vi "xiC - IMAQ - ErrorDialog.vi"(8 "error in (no error)":errorcluster, 11 "Attributes In":T1) -> (0 "error out":errorcluster, 3 "Attributes Out":T1)   [LabVIEW 2013]
uses:
  xiC - IMAQ - Attributes.ctl
  C:/Projects/Cameras3.x/xiLib/xiLIB_64bit/xiLIB/xiCamLib/API/x64/xiApi.NETX64.dll
  xiLIB_64bit/xiLIB/xiCamLib/API/x64/xiApi.NETX64.dll
  xiC - IMAQ - TreeDisplayType.ctl
  xiC - IMAQ - Globals.vi
panel:
  in  "CopyToClipboard":bool
  in  "EXIT":bool
  out "INFO":string
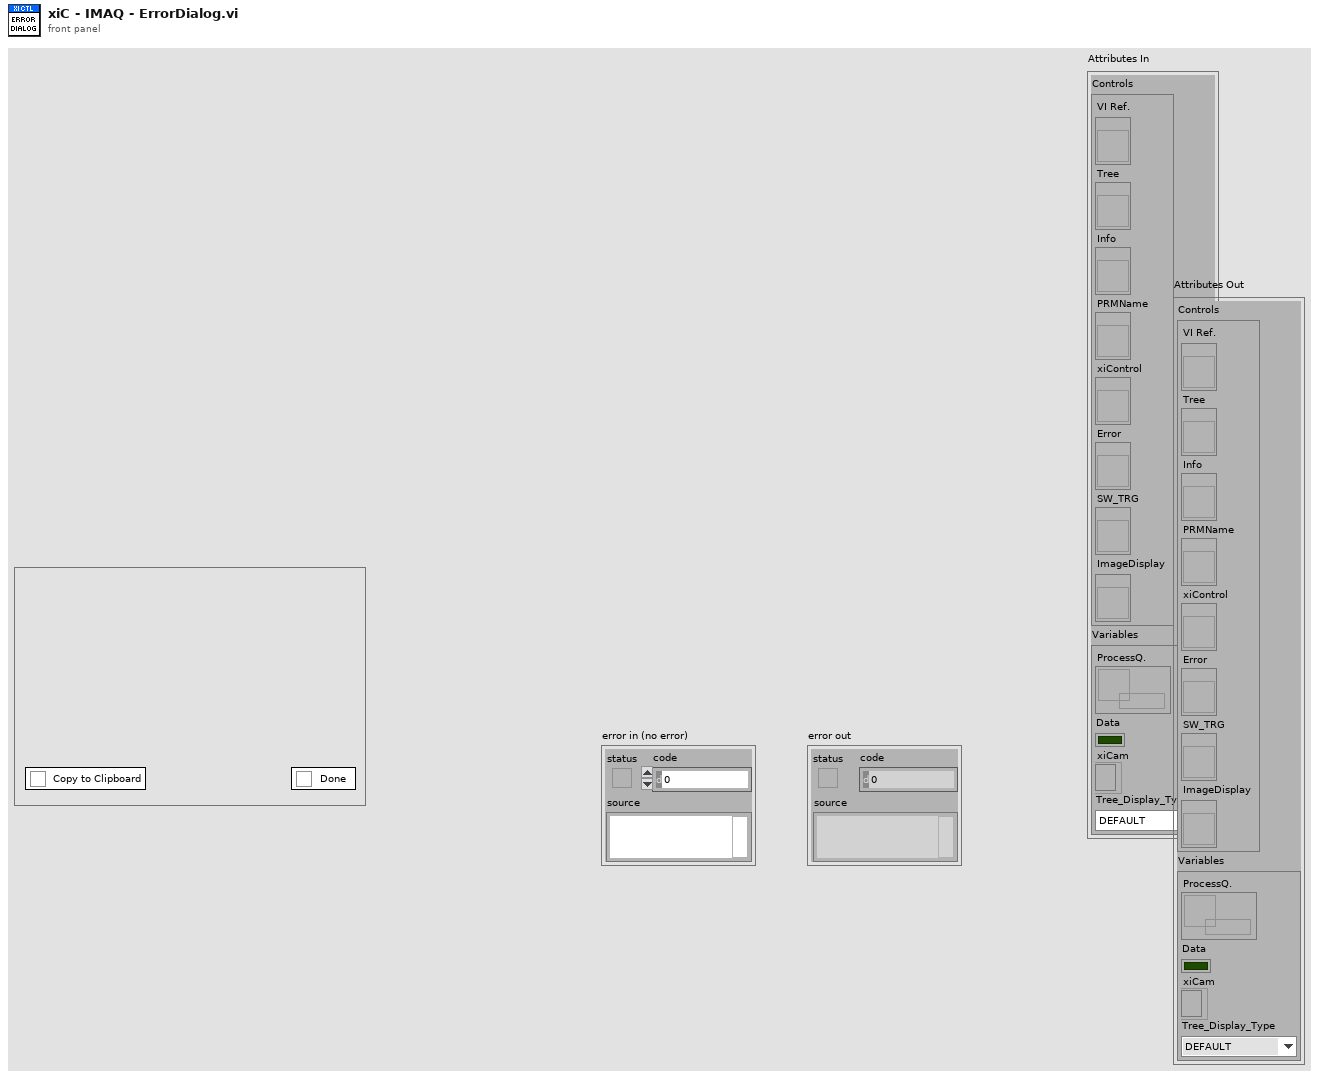
[diagram p1: front panel]
types:
  T1 = typedef "xiC - IMAQ - Attributes.ctl" = cluster{"Controls":cluster{"VI Ref.":refnum<vi>, "Tree":refnum<vi>, "Info":refnum<vi>, "PRMName":refnum<vi>, "xiControl":refnum<vi>, "Error":refnum<vi>, "SW_TRG":refnum<vi>, "ImageDisplay":refnum<vi>}, "Variables":cluster{"ProcessQ.":refnum<queue>, "Data":bool, "xiCam":refnum<k24>, "Tree_Display_Type":T2}}
  T2 = typedef "xiC - IMAQ - TreeDisplayType.ctl" = enum16{"DEFAULT", "HIDE_MAX_MIN"}
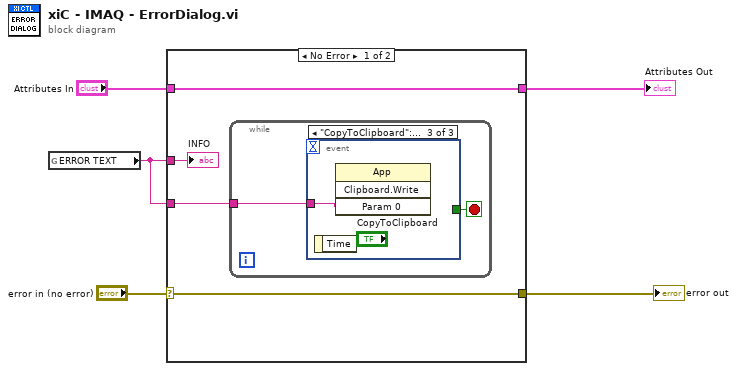
[diagram p0: block diagram]
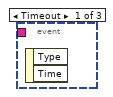
[diagram p2: hidden frame]
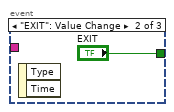
[diagram p3: hidden frame]
diagram:
  n1 = global read "xiC - IMAQ - Globals.vi" "ERROR TEXT"() -> (w1:string)
  n2 = case shown="No Error" "error in (no error)" {
    selector: "error in (no error)" -> [w9 w15]
    tunnel: [w9 w15] -> w4
    tunnel: "Attributes In" -> [w8 w14]
    tunnel: [w8 w14] -> w2
    tunnel: w1 -> [w7 _]
    tunnel: w1 -> [w6 _]
    frame No Error {
      n3 = while {
        tunnel: w6 -> [w10]
        stop <- w11 stop-if-true
        n4 = event shown="[2] \"CopyToClipboard\": Value Change" {
          selector: _ -> [_ _ _]
          dyn-events: _ -> [_ _ _]
          timeout: _ -> [_ _ _]
          tunnel: [_ "EXIT" _] -> w11
          tunnel: w10 -> [_ _ w13]
          event Timeout {
            n5 = event-data() -> ()  [unwired: 1 in, 2 out]
          }
          event "EXIT": Value Change {
            n6 = event-data() -> ()  [unwired: 1 in, 2 out]
          }
          event "CopyToClipboard": Value Change {
            n7 = event-data() -> ()  [unwired: 1 in, 1 out]
            n8 = invoke class="App" method="Clipboard.Write"("Param 0"=w13) -> ()  [unwired: 3 in, 4 out]
          }
        }
      }
      "INFO" <- w7
    }
    frame Error {
    }
  }
  "error out" <- w4
  "Attributes Out" <- w2
